vi "Module Type.vi"(11 "Log Preparer Module in":refnum<class "Log Preparer Module.lvclass">) -> (2 "Module Type":string)   [LabVIEW 2020, in "VolatusData.lvlib" / "Log Preparer Module.lvclass"]
uses:
  Log Preparer Module.lvclass
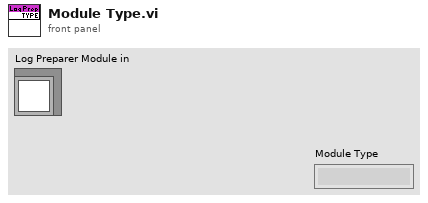
[diagram p1: front panel]
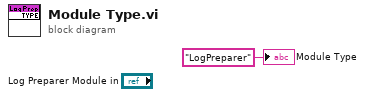
[diagram p0: block diagram]
diagram:
  "Module Type" <- "LogPreparer" ("Module Type")
